vi "RampStateMachine.vi"(8 "error in (no error)":errorcluster) -> (0 "error out":errorcluster)   [LabVIEW 2013]
doc: "Use this template to build a VI to use as a subVI."
uses:
  RampProgramModel/RampProgramModel.lvclass
  RampProgramModel/RampProgramModel.lvclass/RampProgramModel.ctl
  RampState.ctl
  <vilib>/Utility/file.llb/Read From Spreadsheet File (DBL).vi
  <vilib>/Utility/file.llb/Write To Spreadsheet File (string).vi
panel:
  in  "Clear Table":bool
  in  "Repeat Program":u32=1 min=1 max=1000 step=1
  out "Current Repeat":u32=1 min=1 max=1000 step=1
  out "Repeat Program ind":u32=1 min=1 max=1000 step=1
  in  "SaveProgram":bool
  in  "LoadProgram":bool
  in  "PauseProgram":bool
  out "Time Elapsed":dbl
  out "Cooling rate (°C/min)":dbl
  out "SP (°C)":dbl
  in  "StopProgram":bool
  in  "RunProgram":bool
  in  "Current Temperature":dbl(slide) scale=-50.0..20.0 scale format="%.1g"
  out "Status":string
  in  "stop":bool
  in  "Add Entry":bool
  out "Ramp Program Table":string[][](table)
  # "Hardware Abstraction"
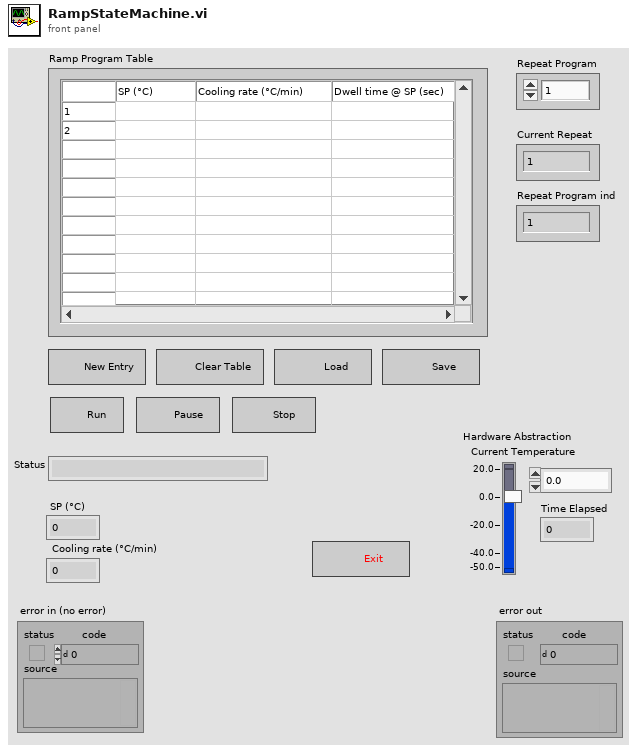
[diagram p1: front panel]
types:
  T1 = typedef "RampState.ctl" = enum16{"Pause Program", "Heatling/Cooling", "Dwelling @ SP", "Stopped"}
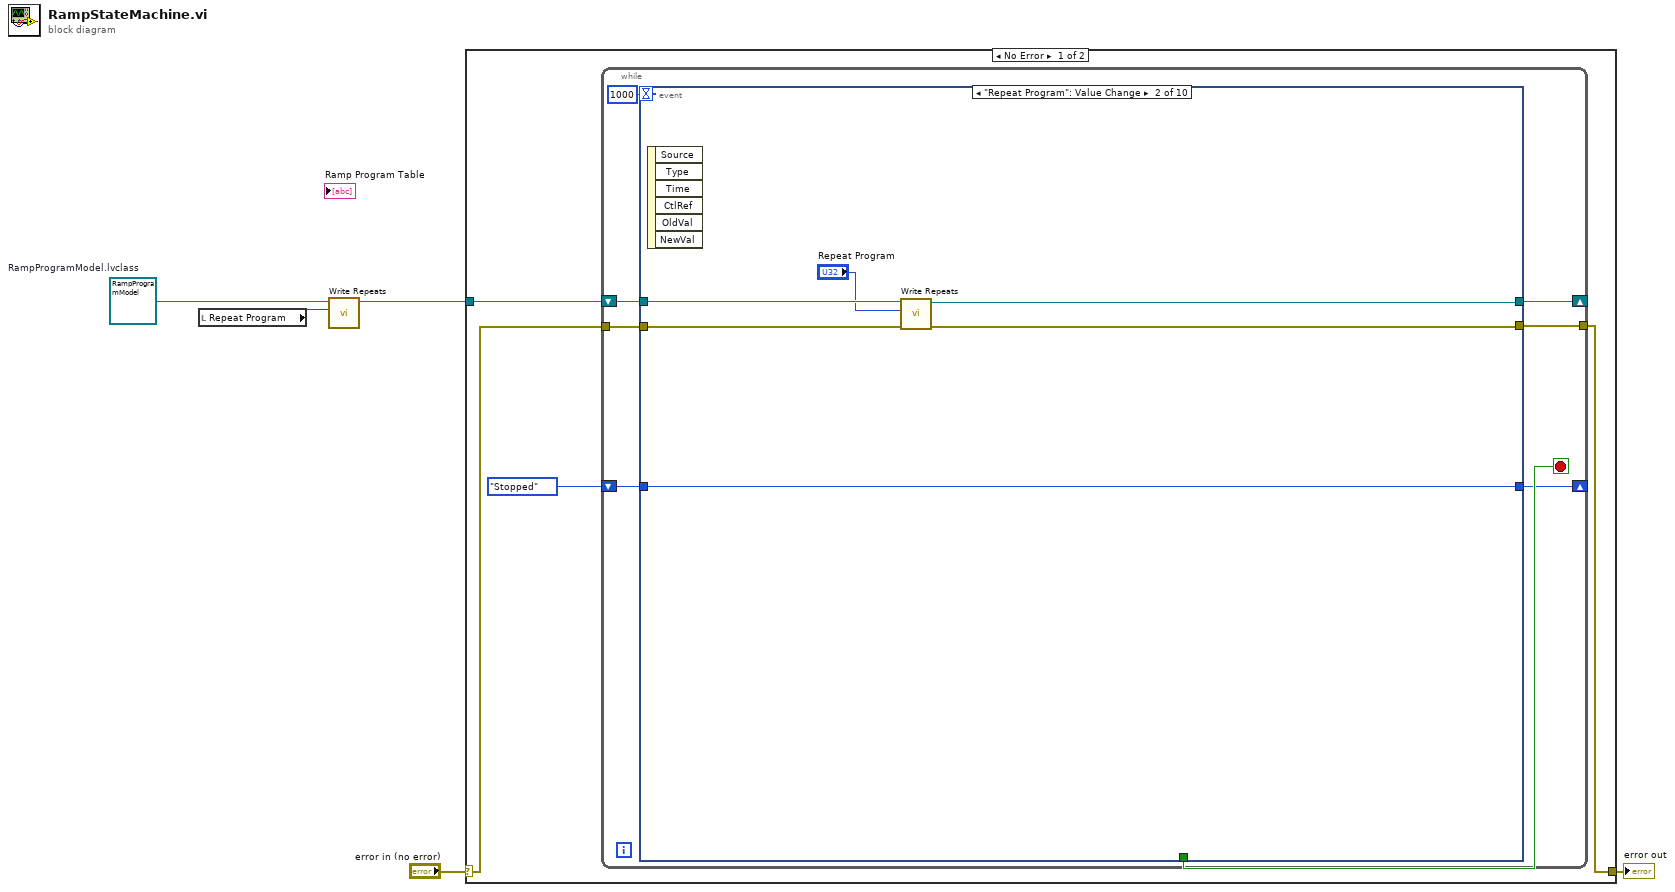
[diagram p0: block diagram]
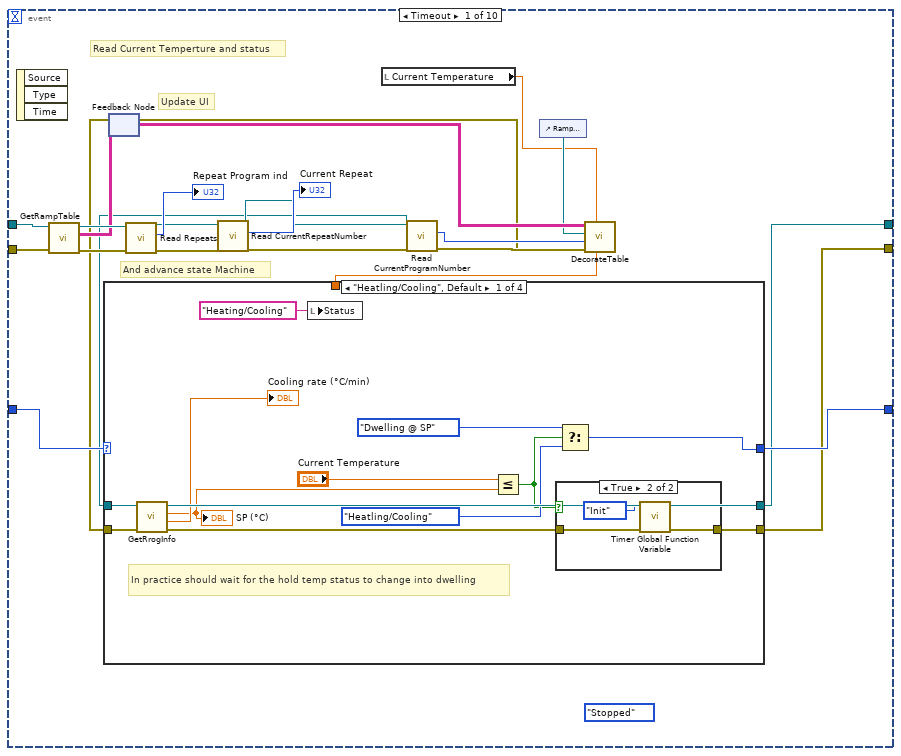
[diagram p2: hidden frame]
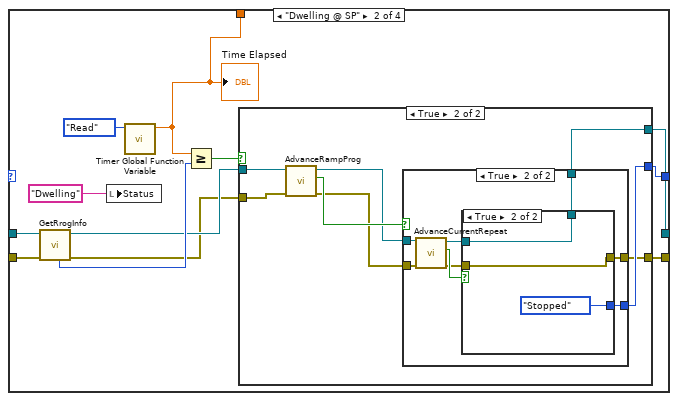
[diagram p4: hidden frame]
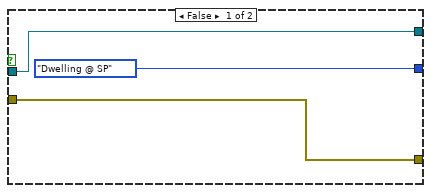
[diagram p5: hidden frame]
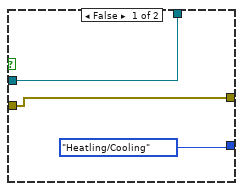
[diagram p6: hidden frame]
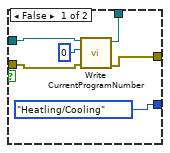
[diagram p7: hidden frame]
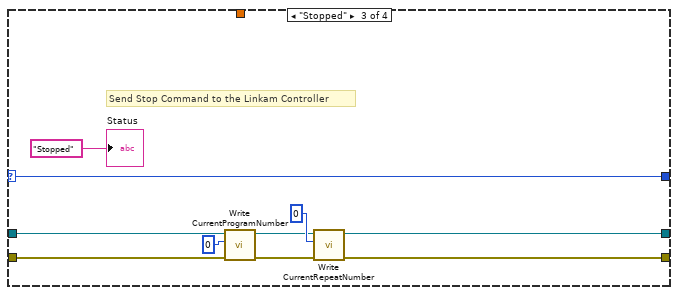
[diagram p8: hidden frame]
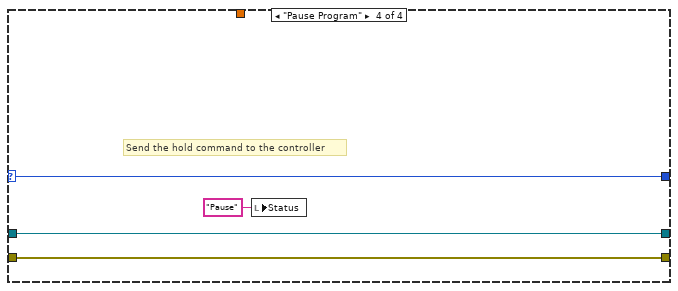
[diagram p9: hidden frame]
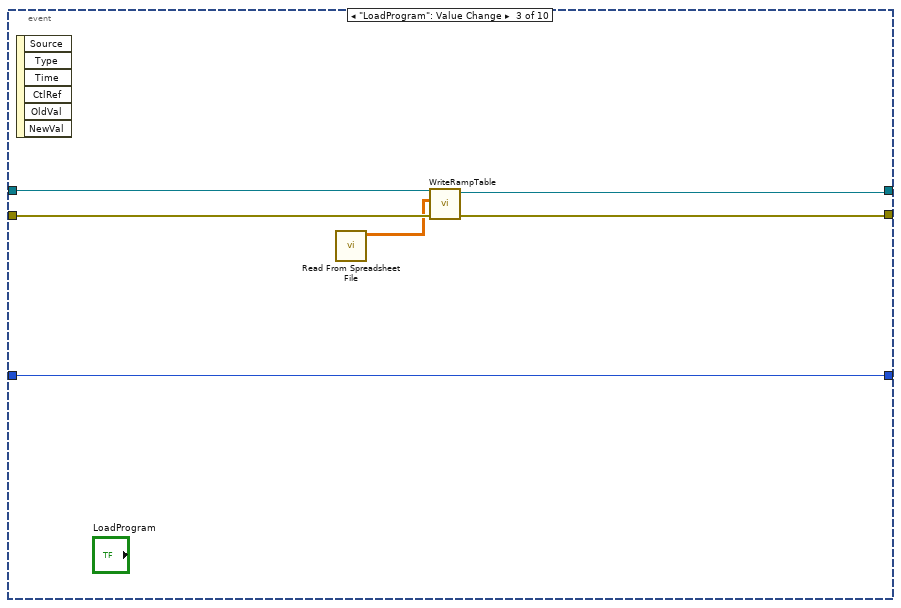
[diagram p10: hidden frame]
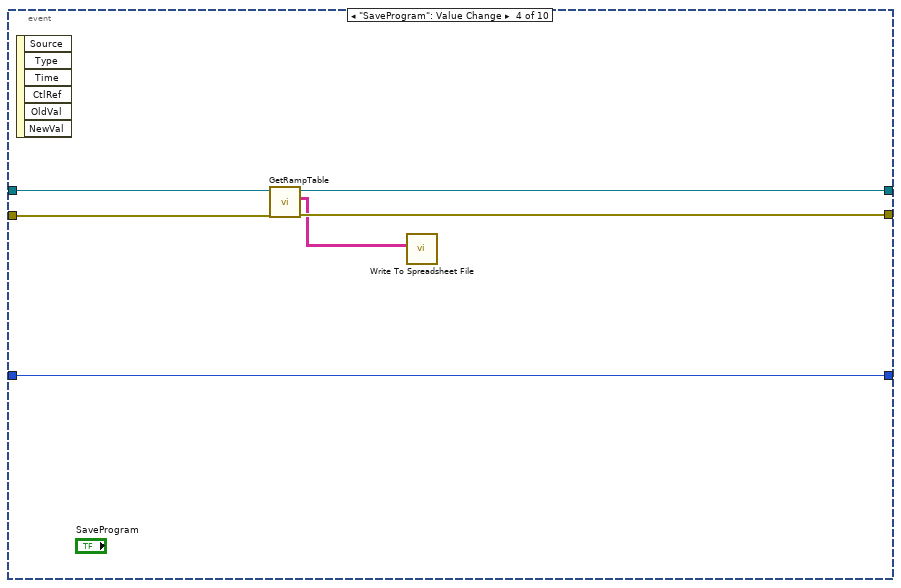
[diagram p11: hidden frame]
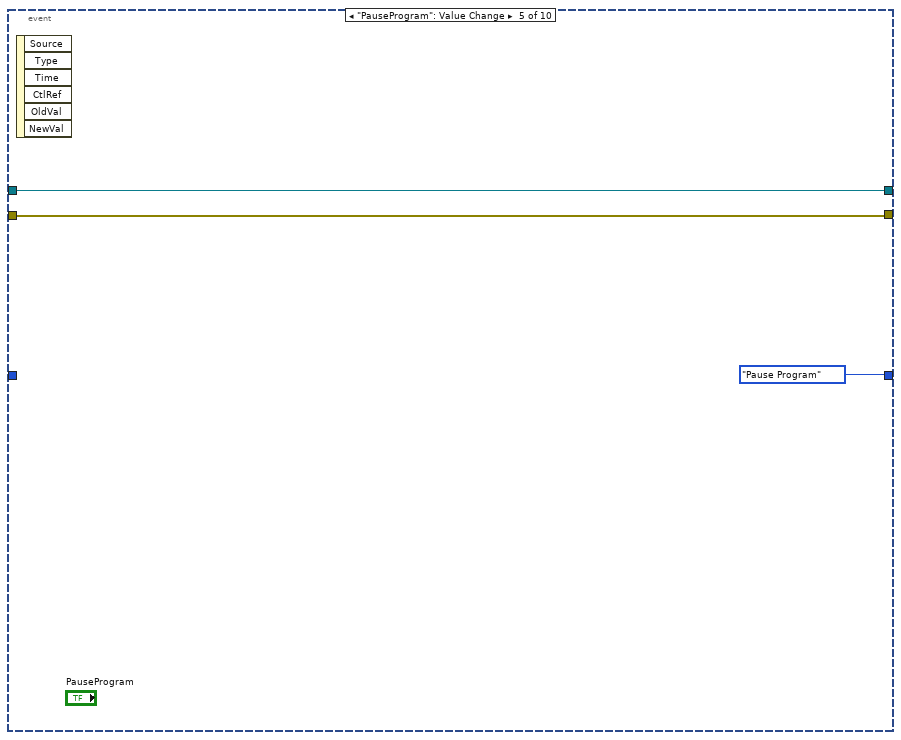
[diagram p12: hidden frame]
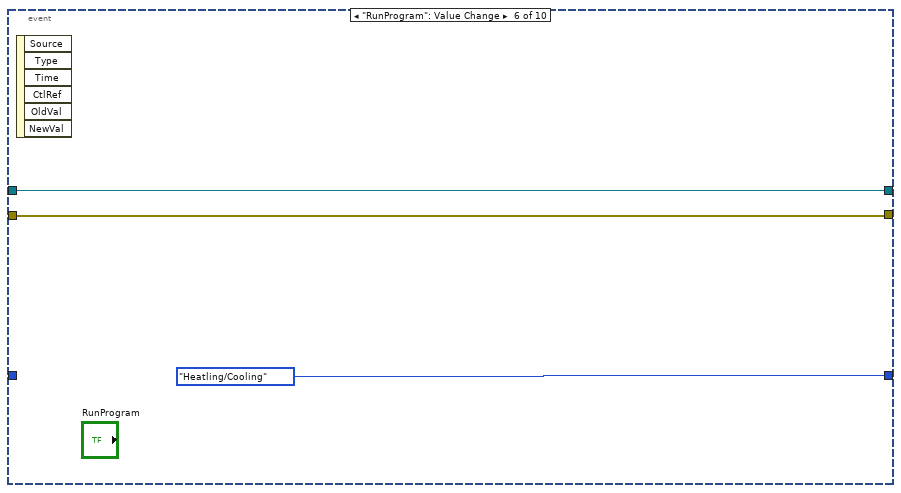
[diagram p13: hidden frame]
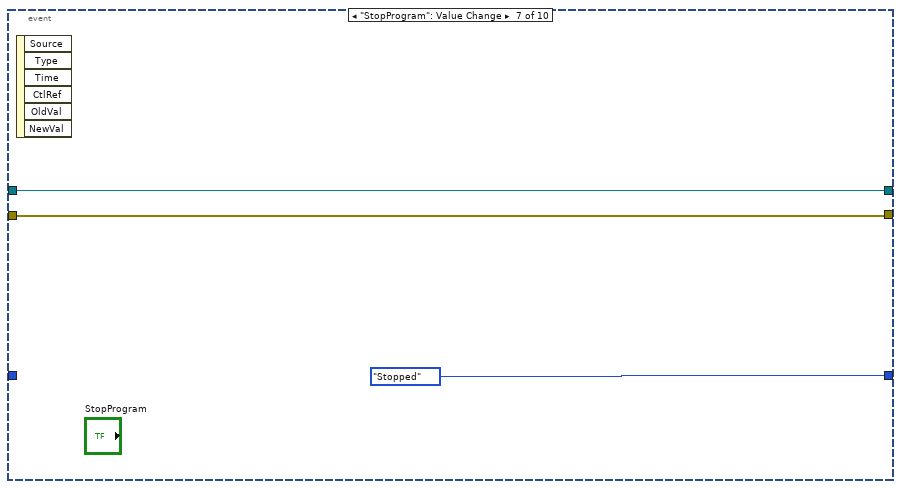
[diagram p14: hidden frame]
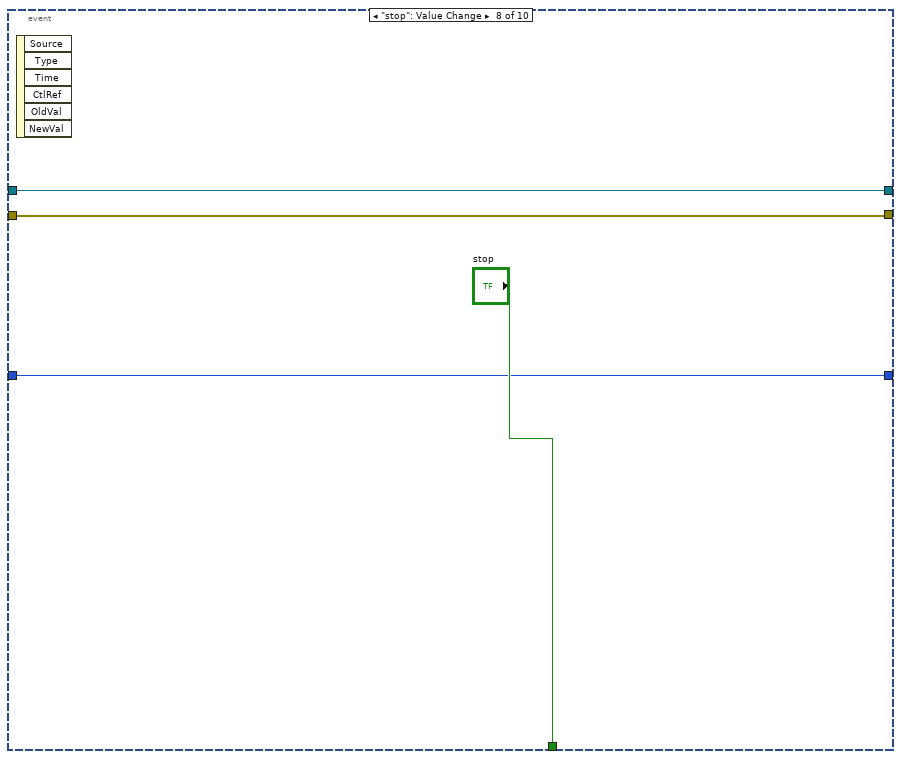
[diagram p15: hidden frame]
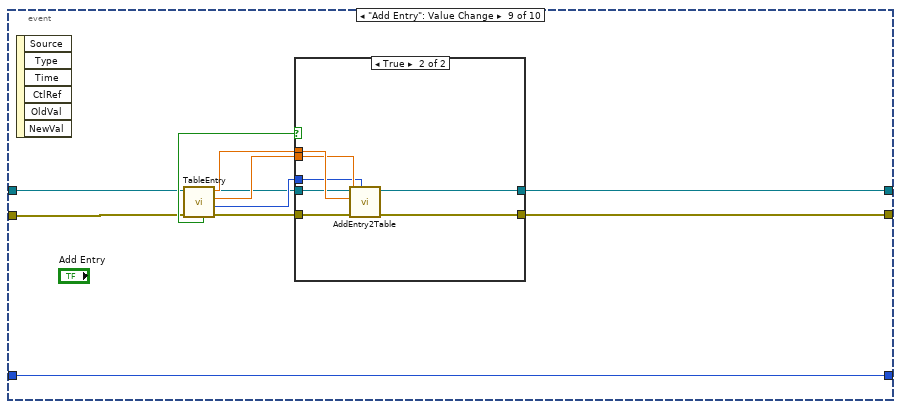
[diagram p16: hidden frame]
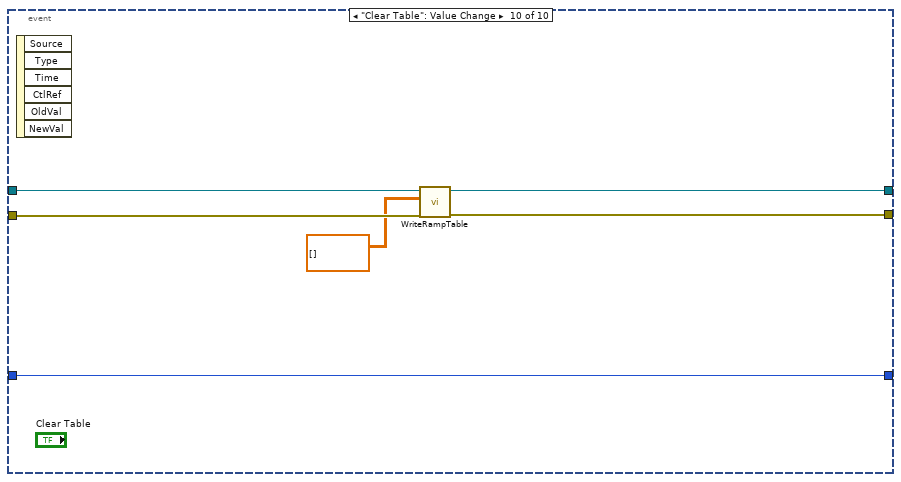
[diagram p18: hidden frame]
diagram:
  w2 = refnum<class "RampProgramModel.lvclass"> refnum  # RampProgramModel.lvclass
  n1 = local read "Repeat Program"() -> (w3:u32)
  n2 = call "Write Repeats.vi"("Repeats"=w3, "RampProgramModel in"=w2) -> ("RampProgramModel out"=w1:refnum<class "RampProgramModel.lvclass">)  [unwired: 8 in, 1 out]
  n3 = case shown="No Error" "error in (no error)" {
    selector: "error in (no error)" -> [w9 w170]
    tunnel: [w8 w170] -> w4
    tunnel: w1 -> [w7 _]
    frame No Error {
      n4 = while {
        tunnel: w9 -> [w16]
        tunnel: [w15] -> w8
        shift-right: [w13] -> _
        shift-left: w7 -> [w14]
        shift-right: [w10] -> _
        shift-left: RampState."Stopped" ("State") -> [w11]
        stop <- w17 stop-if-true
        n5 = event shown="[1] \"Repeat Program\": Value Change" {
          selector: _ -> [_ _ _ _ _ _ _ _ _ _]
          dyn-events: _ -> [_ _ _ _ _ _ _ _ _ _]
          timeout: u32 1000 ("milliseconds to wait") -> [_ _ _ _ _ _ _ _ _ _]
          tunnel: [_ _ _ _ _ _ _ "stop" _ _] -> w17
          tunnel: w16 -> [w40 w119 w124 w129 w133 w135 w139 w143 w153 w167]
          tunnel: [w35 w118 w124 w127 w133 w135 w139 w143 w148 w166] -> w15
          tunnel: w14 -> [w39 w120 w123 w130 w134 w136 w138 w142 w146 w168]
          tunnel: [w36 w117 w122 w128 w134 w136 w138 w142 w147 w165] -> w13
          tunnel: w11 -> [w38 w115 w125 w131 _ _ _ w141 w145 w169]
          tunnel: [w37 w115 w125 w131 RampState."Pause Program" ("State") RampState."Heatling/Cooling" ("State") RampState."Stopped" ("State") w141 w145 w169] -> w10
          event Timeout {
            (unwired) RampState."Stopped" ("State")
            # "Read Current Temperture and status"
            # "And advance state Machine"
            # "Update UI"
            n6 = event-data() -> ()  [unwired: 1 in, 3 out]
            n7 = call "GetRampTable.vi"("error in (no error)"=w40, "RampProgramModel in"=w39) -> ("error out"=w32:errorcluster, "RampTable"=w28:string[][], "RampProgramModel out"=w34:refnum<class "RampProgramModel.lvclass">)  [unwired: 7 in]
            n8 = feedback #1() -> (w18:errorcluster)  [unwired: 1 in]
            n9 = call "Read Repeats.vi"("error in (no error)"=w32, "RampProgramModel in"=w34) -> ("error out"=w30:errorcluster, "Repeats"=→"Repeat Program ind":u32, "RampProgramModel out"=w31:refnum<class "RampProgramModel.lvclass">)  [unwired: 7 in]
            n10 = call "Read CurrentRepeatNumber.vi"("error in (no error)"=w30, "RampProgramModel in"=w31) -> ("error out"=w24:errorcluster, "CurrentRepeatNumber"=→"Current Repeat":u32, "RampProgramModel out"=w25:refnum<class "RampProgramModel.lvclass">)  [unwired: 7 in]
            n11 = local read "Current Temperature"() -> (w21:dbl)
            n12 = call "Read CurrentProgramNumber.vi"("error in (no error)"=w24, "RampProgramModel in"=w25) -> ("error out"=w20:errorcluster, "CurrentProgramNumber"=w22:u32, "RampProgramModel out"=w23:refnum<class "RampProgramModel.lvclass">)  [unwired: 7 in]
            n13 = case shown="\"Heatling/Cooling\", Default" w38 {
              selector: w38 -> [_ _ w110 w112]
              tunnel: [w46 w63 w110 w112] -> w37
              tunnel: w23 -> [w52 w68 w108 w111]
              tunnel: [w51 w60 w101 w111] -> w36
              tunnel: w18 -> [w50 w67 w106 w113]
              tunnel: [w41 w59 w102 w113] -> w35
              tunnel: [_ w58 _ _] -> w26
              frame "Heatling/Cooling", Default {
                # "In practice should wait for the hold temp status to change into dwelling"
                n14 = call "GetRrogInfo.vi"("error in (no error)"=w50, "RampProgramModel in"=w52) -> ("error out"=w42:errorcluster, "Cooling rate (°C/min)"=→"Cooling rate (°C/min)":dbl, "SP (°C)"=w44:dbl, "RampProgramModel out"=w51:refnum<class "RampProgramModel.lvclass">)  [unwired: 5 in, 1 out]
                "SP (°C)" <- w44
                n15 = local write "Status"("Heating/Cooling" ("Status")) -> ()
                n16 = Less Or Equal?(x="Current Temperature", y=w44) -> (x <= y?=w43:bool)
                n17 = case shown="True" w43 {
                  tunnel: w42 -> [w54 w56]
                  tunnel: [w54 w55] -> w41
                  frame False {
                  }
                  frame True {
                    n18 = call "Timer Global Function Variable.vi"("error in (no error)"=w56, "Enum"=enum16{"Init", "Read", "Set"}."Init") -> ("error out"=w55:errorcluster)  [unwired: 7 in, 2 out]
                  }
                }
                n19 = Select(t=RampState."Dwelling @ SP" ("State"), s=w43, f=RampState."Heatling/Cooling" ("State")) -> (s? t:f=w46:T1)
              }
              frame "Dwelling @ SP" {
                n20 = call "GetRrogInfo.vi"("error in (no error)"=w67, "RampProgramModel in"=w68) -> ("error out"=w61:errorcluster, "RampProgramModel out"=w62:refnum<class "RampProgramModel.lvclass">, "Dwell Time @ SP (sec)"=w65:u32)  [unwired: 5 in, 2 out]
                n21 = local write "Status"("Dwelling" ("Status")) -> ()
                n22 = call "Timer Global Function Variable.vi"("Enum"=enum16{"Init", "Read", "Set"}."Read") -> ("Time Elapsed"=w58:dbl)  [unwired: 8 in, 2 out]
                "Time Elapsed" <- w58
                n23 = Greater Or Equal?(x=w58, y=w65) -> (x >= y?=w64:bool)
                n24 = case shown="True" w64 {
                  tunnel: [RampState."Dwelling @ SP" ("State") w75] -> w63
                  tunnel: w62 -> [w71 w80]
                  tunnel: w61 -> [w70 w79]
                  tunnel: [w71 w74] -> w60
                  tunnel: [w70 w73] -> w59
                  frame False {
                  }
                  frame True {
                    n25 = call "AdvanceRampProg.vi"("error in (no error)"=w79, "RampProgramModel in"=w80) -> ("error out"=w76:errorcluster, "EndOfPrograms"=w78:bool, "RampProgramModel out"=w77:refnum<class "RampProgramModel.lvclass">)  [unwired: 7 in]
                    n26 = case shown="True" w78 {
                      tunnel: w77 -> [w81 w91]
                      tunnel: w76 -> [w82 w90]
                      tunnel: [RampState."Heatling/Cooling" ("State") w86] -> w75
                      tunnel: [w81 w85] -> w74
                      tunnel: [w82 w84] -> w73
                      frame False {
                      }
                      frame True {
                        n27 = call "AdvanceCurrentRepeat.vi"("error in (no error)"=w90, "RampProgramModel in"=w91) -> ("error out"=w87:errorcluster, "EndOfRepeats"=w89:bool, "RampProgramModel out"=w88:refnum<class "RampProgramModel.lvclass">)  [unwired: 7 in]
                        n28 = case shown="True" w89 {
                          tunnel: w88 -> [w95 w98]
                          tunnel: w87 -> [w94 w99]
                          tunnel: [RampState."Heatling/Cooling" ("State") RampState."Stopped" ("State")] -> w86
                          tunnel: [w92 w98] -> w85
                          tunnel: [w93 w99] -> w84
                          frame False {
                            n29 = call "Write CurrentProgramNumber.vi"("error in (no error)"=w94, "CurrentProgramNumber"=u32 0, "RampProgramModel in"=w95) -> ("error out"=w93:errorcluster, "RampProgramModel out"=w92:refnum<class "RampProgramModel.lvclass">)  [unwired: 7 in]
                          }
                          frame True {
                          }
                        }
                      }
                    }
                  }
                }
              }
              frame "Stopped" {
                # "Send Stop Command to the Linkam Controller"
                n30 = call "Write CurrentProgramNumber.vi"("error in (no error)"=w106, "CurrentProgramNumber"=u32 0, "RampProgramModel in"=w108) -> ("error out"=w103:errorcluster, "RampProgramModel out"=w104:refnum<class "RampProgramModel.lvclass">)  [unwired: 7 in]
                n31 = call "Write CurrentRepeatNumber.vi"("error in (no error)"=w103, "CurrentRepeatNumber"=u32 0, "RampProgramModel in"=w104) -> ("error out"=w102:errorcluster, "RampProgramModel out"=w101:refnum<class "RampProgramModel.lvclass">)  [unwired: 7 in]
                "Status" <- "Stopped" ("Status")
              }
              frame "Pause Program" {
                # "Send the hold command to the controller"
                n32 = local write "Status"("Pause" ("Status")) -> ()
              }
            }
            n33 = control-ref of="Ramp Program Table"() -> (w27:refnum<vi>)
            n34 = call "DecorateTable.vi"("Elapsed Time"=w26, "Current Temperature"=w21, "error in (no error)"=w20, "Current Program"=w22, "Tbl Refnum"=w27, "RampTable"=w28) -> ("error out"=w19:errorcluster)  [unwired: 5 in]
            n35 = feedback-in #1(w19) -> ()
          }
          event "Repeat Program": Value Change {
            n36 = event-data() -> ()  [unwired: 1 in, 6 out]
            n37 = call "Write Repeats.vi"("error in (no error)"=w119, "Repeats"="Repeat Program", "RampProgramModel in"=w120) -> ("error out"=w118:errorcluster, "RampProgramModel out"=w117:refnum<class "RampProgramModel.lvclass">)  [unwired: 7 in]
          }
          event "LoadProgram": Value Change {
            n38 = event-data() -> ()  [unwired: 1 in, 6 out]
            n39 = call-poly <vilib>:"Read From Spreadsheet File.vi"() -> ("all rows"=w121:dbl[][])  [unwired: 7 in, 4 out]
            n40 = call "WriteRampTable.vi"("RampFromFile"=w121, "RampProgramModel in"=w123) -> ("RampProgramModel out"=w122:refnum<class "RampProgramModel.lvclass">)  [unwired: 8 in, 1 out]
          }
          event "SaveProgram": Value Change {
            n41 = event-data() -> ()  [unwired: 1 in, 6 out]
            n42 = call "GetRampTable.vi"("error in (no error)"=w129, "RampProgramModel in"=w130) -> ("error out"=w127:errorcluster, "RampTable"=w126:string[][], "RampProgramModel out"=w128:refnum<class "RampProgramModel.lvclass">)  [unwired: 7 in]
            n43 = call-poly <vilib>:"Write To Spreadsheet File.vi"("2D data"=w126) -> ()  [unwired: 7 in, 1 out]
          }
          event "PauseProgram": Value Change {
            n44 = event-data() -> ()  [unwired: 1 in, 6 out]
          }
          event "RunProgram": Value Change {
            n45 = event-data() -> ()  [unwired: 1 in, 6 out]
          }
          event "StopProgram": Value Change {
            n46 = event-data() -> ()  [unwired: 1 in, 6 out]
          }
          event "stop": Value Change {
            n47 = event-data() -> ()  [unwired: 1 in, 6 out]
          }
          event "Add Entry": Value Change {
            n48 = event-data() -> ()  [unwired: 1 in, 6 out]
            n49 = call "TableEntry.vi"("error in (no error)"=w153) -> ("error out"=w149:errorcluster, "Dwell Time @ SP (sec) 2"=w150:u32, "Cooling rate (°C/min) 2"=w151:dbl, "SP (°C) 2"=w152:dbl, "Add Entry Pressed?"=w154:bool)  [unwired: 6 in]
            n50 = case shown="True" w154 {
              tunnel: w152 -> [_ w163]
              tunnel: w151 -> [_ w162]
              tunnel: w150 -> [_ w161]
              tunnel: w149 -> [w156 w160]
              tunnel: [w156 w157] -> w148
              tunnel: w146 -> [w155 w159]
              tunnel: [w155 w158] -> w147
              frame False {
              }
              frame True {
                n51 = call "AddEntry2Table.vi"("Dwell Time @ SP (sec)"=w161, "error in (no error)"=w160, "Cooling rate (°C/min)"=w162, "SP (°C)"=w163, "RampProgramModel in"=w159) -> ("error out"=w157:errorcluster, "RampProgramModel out"=w158:refnum<class "RampProgramModel.lvclass">)  [unwired: 5 in]
              }
            }
          }
          event "Clear Table": Value Change {
            n52 = event-data() -> ()  [unwired: 1 in, 6 out]
            n53 = call "WriteRampTable.vi"("error in (no error)"=w167, "RampFromFile"=dbl[][] [], "RampProgramModel in"=w168) -> ("error out"=w166:errorcluster, "RampProgramModel out"=w165:refnum<class "RampProgramModel.lvclass">)  [unwired: 7 in]
          }
        }
      }
    }
    frame Error {
    }
  }
  "error out" <- w4
